vi "Wash Display Console View.vi"(8 "error in (no error)":errorcluster, 11 "View Model":T2) -> (0 "error out":errorcluster)   [LabVIEW 2017]
doc: "The interface via which the wash controller displays the progress of the car wash.\n[Covers: UI3]"
uses:
  View Model/Controls/View Model.ctl
  View Model/Controls/Shared Model.ctl
  Error Handler/Controls/Error Model.ctl
  Error Handler/Controls/Error Message.ctl
  Error Handler/Controls/Error Level.ctl
  Configuration/Controls/Database Model.ctl
  Configuration/Controls/Database Message.ctl
  Configuration/Controls/Database Command.ctl
  Configuration/Controls/Database Overhead.ctl
  Configuration/Controls/Database Status.ctl
  Configuration/Controls/Database Record.ctl
  Configuration/Controls/Database - Rule Record.ctl
  Controller/Controls/CNTRLR - Wash Step.ctl
  Controller/Controls/CNTRLR - Position.ctl
  Controller/Controls/CNTRLR - Model.ctl
  Controller/Controls/CNTRLR - Message.ctl
  Controller/Controls/CNTRLR - Command.ctl
  Controller/Controls/CNTRLR - Overhead.ctl
  Controller/Controls/CNTRLR - State.ctl
  Controls/Display - Wash LEDs.ctl
  Controls/Display - UI References.ctl
  Controller/Controls/CNTRLR - Timer CMD.ctl
panel:
  out "Time Remaining":dbl format="%07.2f"
  out "Out of Position":bool caption="Vehicle Out of Position"
  out "Wash Entry":bool
  out "Wash LEDs":T1 caption="Car Wash Indicators"
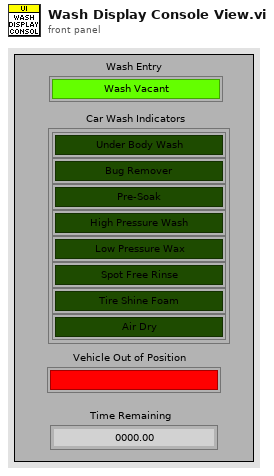
[diagram p1: front panel]
types:
  T1 = typedef "Display - Wash LEDs.ctl" = cluster{"Under Body Wash":bool, "Bug Remover":bool, "Pre-Soak":bool, "High Pressure Wash":bool, "Low Pressure Wax":bool, "Spot Free Rinse":bool, "Tire Shine Foam":bool, "Air Dry":bool}
  T2 = typedef "View Model.ctl" = cluster{"Shared Model":T3, "Error Model":T4, "DB Model":T5, "CNTRLR Model":T6}
  T3 = typedef "Shared Model.ctl" = cluster{"Stop":refnum<user-event>, "Stop DVR":refnum<data-value>}
  T4 = typedef "Error Model.ctl" = cluster{"Error Message":refnum<user-event>}
  T5 = typedef "Database Model.ctl" = cluster{"DB Message":refnum<user-event>, "DB Overhead DVR":refnum<data-value>}
  T6 = typedef "CNTRLR - Model.ctl" = cluster{"Message":refnum<user-event>, "Overhead DVR":refnum<data-value>, "Wash Entry":refnum<user-event>, "Out of Position":refnum<user-event>}
  T7 = typedef "Display - UI References.ctl" = cluster{"Wash Entry":refnum<vi>, "Wash LEDs":refnum<vi>, "Out of Position":refnum<vi>, "Time Remaining":refnum<vi>}
  T8 = typedef "CNTRLR - Timer CMD.ctl" = enum16{"Start", "Get Time", "Pause", "Unpause"}
  T9 = typedef "CNTRLR - State.ctl" = enum16{"Initial", "Wait for Start", "Start State", "Wait for Vehicle Position", "Wash Step Execution", "Wash Step/Cycle Complete", "Wash Exit", "Wash Abort/Terminate"}
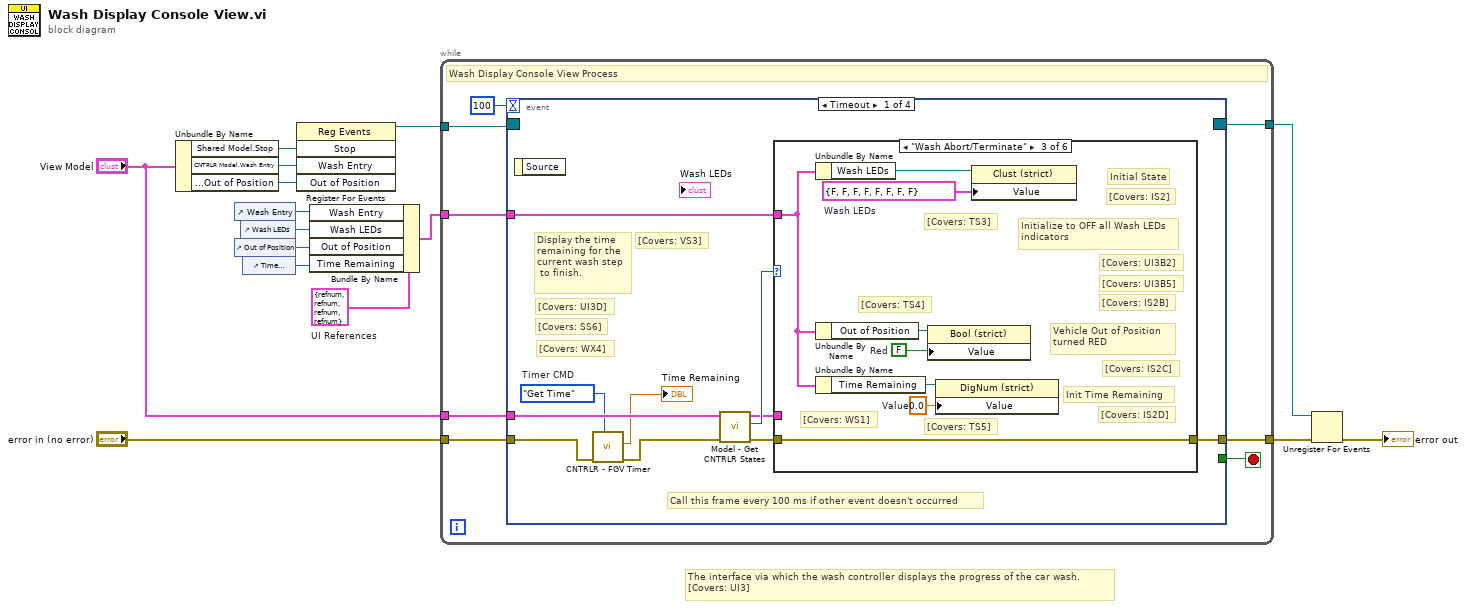
[diagram p0: block diagram]
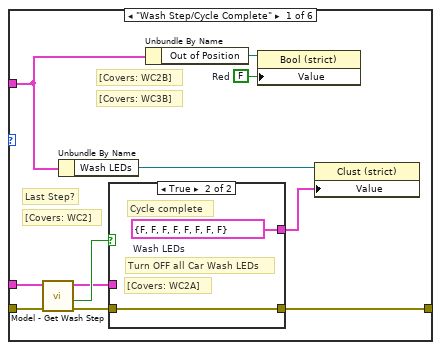
[diagram p2: hidden frame]
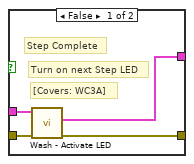
[diagram p3: hidden frame]
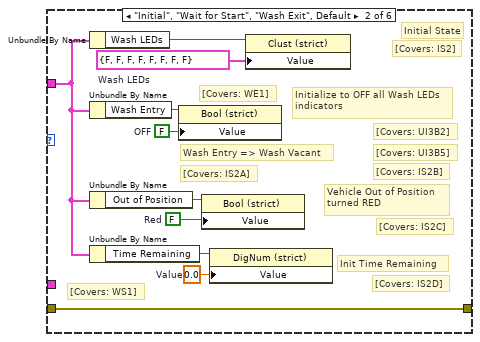
[diagram p4: hidden frame]
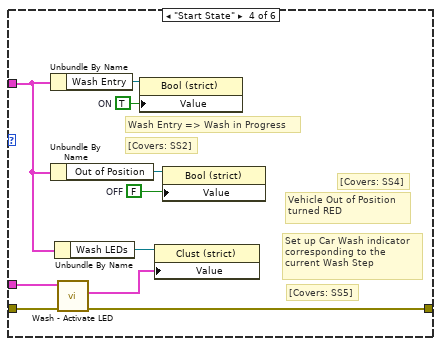
[diagram p5: hidden frame]
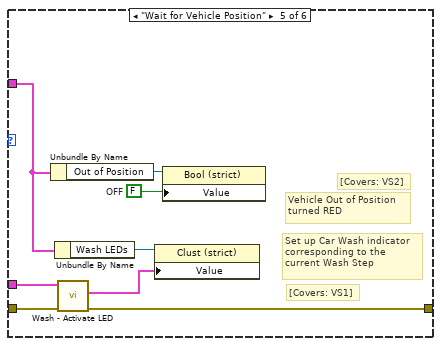
[diagram p6: hidden frame]
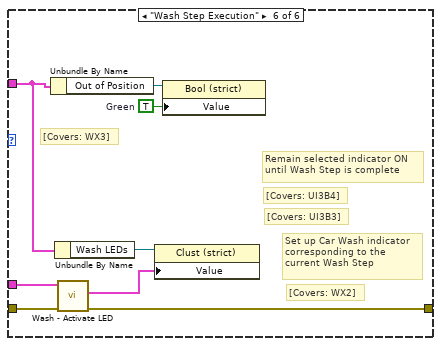
[diagram p7: hidden frame]
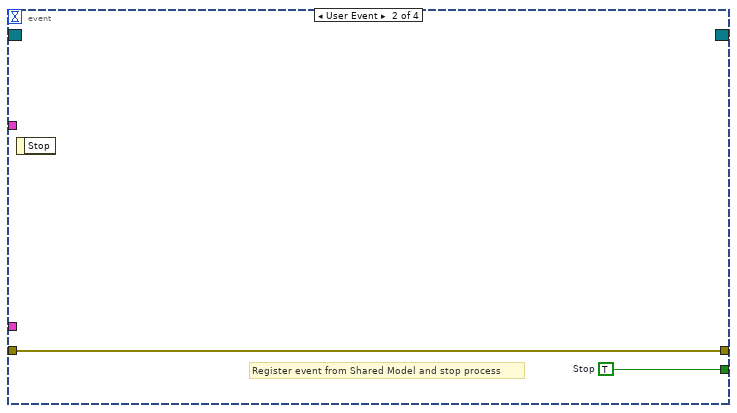
[diagram p8: hidden frame]
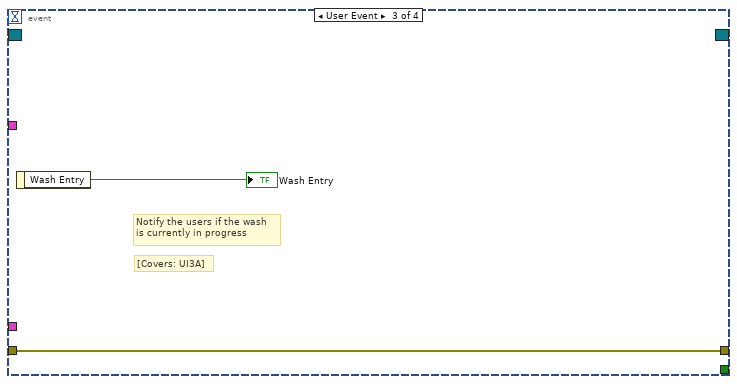
[diagram p9: hidden frame]
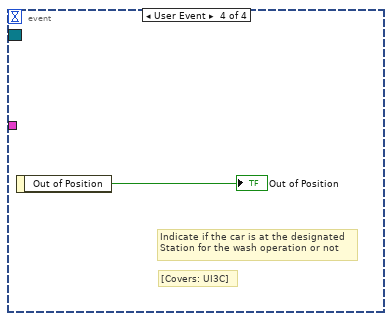
[diagram p10: hidden frame]
diagram:
  w8 = T7 {"Wash Entry"=refnum, "Wash LEDs"=refnum, "Out of Position"=refnum, "Time Remaining"=refnum}  # UI References
  # "The interface via which the wash controller displays the progress of the car wash.\n[Covers: UI3]"
  n1 = Unbundle By Name("View Model") -> ("Shared Model.Stop"=w15:refnum<user-event>, "CNTRLR Model.Wash Entry"=w2:refnum<user-event>, "CNTRLR Model.Out of Position"=w1:refnum<user-event>)
  n2 = control-ref of="Wash Entry"() -> (w7:refnum<vi>)
  n3 = control-ref of="Out of Position"() -> (w5:refnum<vi>)
  n4 = control-ref of="Wash LEDs"() -> (w6:refnum<vi>)
  n5 = control-ref of="Time Remaining"() -> (w4:refnum<vi>)
  n6 = register-events(w15, w2, w1) -> (reference out=w14:refnum<event-registration>)  [unwired: 2 in, 1 out]
  n7 = Bundle By Name(cluster=w8, "Wash Entry"=w7, "Wash LEDs"=w6, "Out of Position"=w5, "Time Remaining"=w4) -> (w3:T7)
  n8 = while {
    tunnel: w14 -> [w23]
    tunnel: "error in (no error)" -> [w22]
    tunnel: [w21] -> w12
    tunnel: [w18] -> w13
    tunnel: "View Model" -> [w17]
    tunnel: w3 -> [w16]
    stop <- w19 stop-if-true
    # "Wash Display Console View Process"
    n9 = event shown="[0] Timeout" {
      selector: w23 -> [_ _ _ _]
      dyn-events: [_ _ _ _] -> w18
      timeout: 100 -> [_ _ _ _]
      tunnel: w22 -> [w28 w95 w98 _]
      tunnel: [w29 w95 w98 _] -> w21
      tunnel: [_ w96 _ _] -> w19
      tunnel: w17 -> [w26 _ _ _]
      tunnel: w16 -> [w32 _ _ _]
      event Timeout {
        w24 = CNTRLR_-_Timer_CMD."Get Time"  # Timer CMD
        # "[Covers: WX4]"
        # "[Covers: VS3]"
        # "[Covers: SS6]"
        # "Display the time\nremaining for the\ncurrent wash step\n to finish."
        # "[Covers: UI3D]"
        # "Call this frame every 100 ms if other event doesn't occurred"
        n10 = event-data() -> ()  [unwired: 1 in, 1 out]
        n11 = call "CNTRLR - FGV Timer.vi"("Timer CMD"=w24, "error in (no error)"=w28) -> ("error out"=w27:errorcluster, "Elapsed Time"=→"Time Remaining":dbl)  [unwired: 7 in, 1 out]
        n12 = call "Model - Get CNTRLR States.vi"("error in (no error)"=w27, "View Model"=w26) -> ("error out"=w31:errorcluster, "Current State"=w33:T9, "View Model"=w30:T2)  [unwired: 6 in, 1 out]
        n13 = case shown="\"Wash Abort/Terminate\"" w33 {
          tunnel: w32 -> [w38 w53 w63 w73 w83 w88]
          tunnel: w31 -> [w43 w58 w66 w72 w82 w93]
          tunnel: w30 -> [w42 _ _ w71 w81 w92]
          tunnel: [w34 w58 w66 w69 w79 w90] -> w29
          frame "Wash Step/Cycle Complete" {
            w39 = FALSE  # Red
            # "[Covers: WC3B]"
            # "[Covers: WC2B]"
            # "Last Step?"
            # "[Covers: WC2]"
            n14 = call "Model - Get Wash Step.vi"("error in (no error)"=w43, "View Model"=w42) -> ("error out"=w37:errorcluster, "Last Step?"=w41:bool, "View Model"=w36:T2)  [unwired: 6 in, 1 out]
            n15 = Unbundle By Name(w38) -> ("Wash LEDs"=w44:refnum<vi>)
            n16 = case shown="True" w41 {
              tunnel: [w46 w50] -> w35
              tunnel: w37 -> [w48 w49]
              tunnel: w36 -> [w47 _]
              tunnel: [w45 w49] -> w34
              frame False {
                # "[Covers: WC3A]"
                # "Turn on next Step LED"
                # "Step Complete"
                n17 = call "Wash - Activate LED.vi"("error in (no error)"=w48, "View Model"=w47) -> ("error out"=w45:errorcluster, "Wash LEDs"=w46:T1)  [unwired: 7 in, 1 out]
              }
              frame True {
                w50 = T1 {"Under Body Wash"=FALSE, "Bug Remover"=FALSE, "Pre-Soak"=FALSE, "High Pressure Wash"=FALSE, "Low Pressure Wax"=FALSE, "Spot Free Rinse"=FALSE, "Tire Shine Foam"=FALSE, "Air Dry"=FALSE}  # Wash LEDs
                # "Turn OFF all Car Wash LEDs"
                # "[Covers: WC2A]"
                # "Cycle complete"
              }
            }
            n18 = Unbundle By Name(w38) -> ("Out of Position"=w40:refnum<vi>)
            n19 = property class="Bool (strict)"(reference=w40, "Value"=w39) -> ()  [unwired: 1 in, 2 out]
            n20 = property class="Clust (strict)"(reference=w44, "Value"=w35) -> ()  [unwired: 1 in, 2 out]
          }
          frame "Initial", "Wait for Start", "Wash Exit", Default {
            w51 = 0.0  # Value
            w54 = FALSE  # Red
            w56 = FALSE  # OFF
            w59 = T1 {"Under Body Wash"=FALSE, "Bug Remover"=FALSE, "Pre-Soak"=FALSE, "High Pressure Wash"=FALSE, "Low Pressure Wax"=FALSE, "Spot Free Rinse"=FALSE, "Tire Shine Foam"=FALSE, "Air Dry"=FALSE}  # Wash LEDs
            # "[Covers: WE1]"
            # "[Covers: WS1]"
            # "[Covers: IS2D]"
            # "Init Time Remaining"
            # "[Covers: IS2C]"
            # "Vehicle Out of Position\nturned RED"
            # "[Covers: IS2A]"
            # "Wash Entry => Wash Vacant"
            # "[Covers: IS2]"
            # "Initial State"
            # "[Covers: IS2B]"
            # "[Covers: UI3B5]"
            # "Initialize to OFF all Wash LEDs\nindicators"
            # "[Covers: UI3B2]"
            n21 = Unbundle By Name(w53) -> ("Wash LEDs"=w60:refnum<vi>)
            n22 = Unbundle By Name(w53) -> ("Wash Entry"=w57:refnum<vi>)
            n23 = Unbundle By Name(w53) -> ("Out of Position"=w55:refnum<vi>)
            n24 = Unbundle By Name(w53) -> ("Time Remaining"=w52:refnum<vi>)
            n25 = property class="Bool (strict)"(reference=w57, "Value"=w56) -> ()  [unwired: 1 in, 2 out]
            n26 = property class="Bool (strict)"(reference=w55, "Value"=w54) -> ()  [unwired: 1 in, 2 out]
            n27 = property class="DigNum (strict)"(reference=w52, "Value"=w51) -> ()  [unwired: 1 in, 2 out]
            n28 = property class="Clust (strict)"(reference=w60, "Value"=w59) -> ()  [unwired: 1 in, 2 out]
          }
          frame "Wash Abort/Terminate" {
            w61 = 0.0  # Value
            w64 = FALSE  # Red
            w67 = T1 {"Under Body Wash"=FALSE, "Bug Remover"=FALSE, "Pre-Soak"=FALSE, "High Pressure Wash"=FALSE, "Low Pressure Wax"=FALSE, "Spot Free Rinse"=FALSE, "Tire Shine Foam"=FALSE, "Air Dry"=FALSE}  # Wash LEDs
            # "[Covers: TS5]"
            # "[Covers: TS4]"
            # "[Covers: TS3]"
            # "[Covers: WS1]"
            # "[Covers: IS2D]"
            # "Init Time Remaining"
            # "[Covers: IS2C]"
            # "Vehicle Out of Position\nturned RED"
            # "[Covers: IS2]"
            # "Initial State"
            # "[Covers: IS2B]"
            # "[Covers: UI3B5]"
            # "Initialize to OFF all Wash LEDs\nindicators"
            # "[Covers: UI3B2]"
            n29 = Unbundle By Name(w63) -> ("Wash LEDs"=w68:refnum<vi>)
            n30 = Unbundle By Name(w63) -> ("Out of Position"=w65:refnum<vi>)
            n31 = Unbundle By Name(w63) -> ("Time Remaining"=w62:refnum<vi>)
            n32 = property class="Bool (strict)"(reference=w65, "Value"=w64) -> ()  [unwired: 1 in, 2 out]
            n33 = property class="DigNum (strict)"(reference=w62, "Value"=w61) -> ()  [unwired: 1 in, 2 out]
            n34 = property class="Clust (strict)"(reference=w68, "Value"=w67) -> ()  [unwired: 1 in, 2 out]
          }
          frame "Start State" {
            w74 = FALSE  # OFF
            w76 = TRUE  # ON
            # "[Covers: SS5]"
            # "Set up Car Wash indicator\ncorresponding to the\ncurrent Wash Step"
            # "[Covers: SS4]"
            # "Vehicle Out of Position\nturned RED"
            # "[Covers: SS2]"
            # "Wash Entry => Wash in Progress"
            n35 = Unbundle By Name(w73) -> ("Wash Entry"=w77:refnum<vi>)
            n36 = Unbundle By Name(w73) -> ("Out of Position"=w75:refnum<vi>)
            n37 = Unbundle By Name(w73) -> ("Wash LEDs"=w78:refnum<vi>)
            n38 = call "Wash - Activate LED.vi"("error in (no error)"=w72, "View Model"=w71) -> ("error out"=w69:errorcluster, "Wash LEDs"=w70:T1)  [unwired: 7 in, 1 out]
            n39 = property class="Bool (strict)"(reference=w77, "Value"=w76) -> ()  [unwired: 1 in, 2 out]
            n40 = property class="Clust (strict)"(reference=w78, "Value"=w70) -> ()  [unwired: 1 in, 2 out]
            n41 = property class="Bool (strict)"(reference=w75, "Value"=w74) -> ()  [unwired: 1 in, 2 out]
          }
          frame "Wait for Vehicle Position" {
            w84 = FALSE  # OFF
            # "[Covers: VS1]"
            # "Set up Car Wash indicator\ncorresponding to the\ncurrent Wash Step"
            # "[Covers: VS2]"
            # "Vehicle Out of Position\nturned RED"
            n42 = Unbundle By Name(w83) -> ("Out of Position"=w85:refnum<vi>)
            n43 = Unbundle By Name(w83) -> ("Wash LEDs"=w86:refnum<vi>)
            n44 = call "Wash - Activate LED.vi"("error in (no error)"=w82, "View Model"=w81) -> ("error out"=w79:errorcluster, "Wash LEDs"=w80:T1)  [unwired: 7 in, 1 out]
            n45 = property class="Clust (strict)"(reference=w86, "Value"=w80) -> ()  [unwired: 1 in, 2 out]
            n46 = property class="Bool (strict)"(reference=w85, "Value"=w84) -> ()  [unwired: 1 in, 2 out]
          }
          frame "Wash Step Execution" {
            w87 = TRUE  # Green
            # "[Covers: WX3]"
            # "[Covers: UI3B4]"
            # "Remain selected indicator ON\nuntil Wash Step is complete"
            # "[Covers: UI3B3]"
            # "[Covers: WX2]"
            # "Set up Car Wash indicator\ncorresponding to the\ncurrent Wash Step"
            n47 = Unbundle By Name(w88) -> ("Out of Position"=w89:refnum<vi>)
            n48 = Unbundle By Name(w88) -> ("Wash LEDs"=w94:refnum<vi>)
            n49 = call "Wash - Activate LED.vi"("error in (no error)"=w93, "View Model"=w92) -> ("error out"=w90:errorcluster, "Wash LEDs"=w91:T1)  [unwired: 7 in, 1 out]
            n50 = property class="Clust (strict)"(reference=w94, "Value"=w91) -> ()  [unwired: 1 in, 2 out]
            n51 = property class="Bool (strict)"(reference=w89, "Value"=w87) -> ()  [unwired: 1 in, 2 out]
          }
        }
      }
      event User Event {
        w96 = TRUE  # Stop
        # "Register event from Shared Model and stop process"
        n52 = event-data() -> ()  [unwired: 1 in, 1 out]
      }
      event User Event {
        # "[Covers: UI3A]"
        # "Notify the users if the wash\nis currently in progress"
        n53 = event-data() -> ("Wash Entry"=→"Wash Entry":bool)  [unwired: 1 in]
      }
      event User Event {
        # "[Covers: UI3C]"
        # "Indicate if the car is at the designated\nStation for the wash operation or not"
        n54 = event-data() -> ("Out of Position"=→"Out of Position":bool)  [unwired: 1 in]
      }
    }
  }
  n55 = Unregister For Events(event registration refnum=w13, error in=w12) -> (error out=→"error out":errorcluster)
